vi "Split.vi"(2 "error in":errorcluster caption="错误输入（无错误）", 3 "ViewCtl":T1) -> (0 "error out":errorcluster caption="错误输出", 1 "StartArr":bool[](array[boolean]))   [LabVIEW 2013]
uses:
  Ctl/ViewCtl.ctl
  USBCAN/DevType.ctl
panel:
  # "ms"
  # "ms"
  # "s"
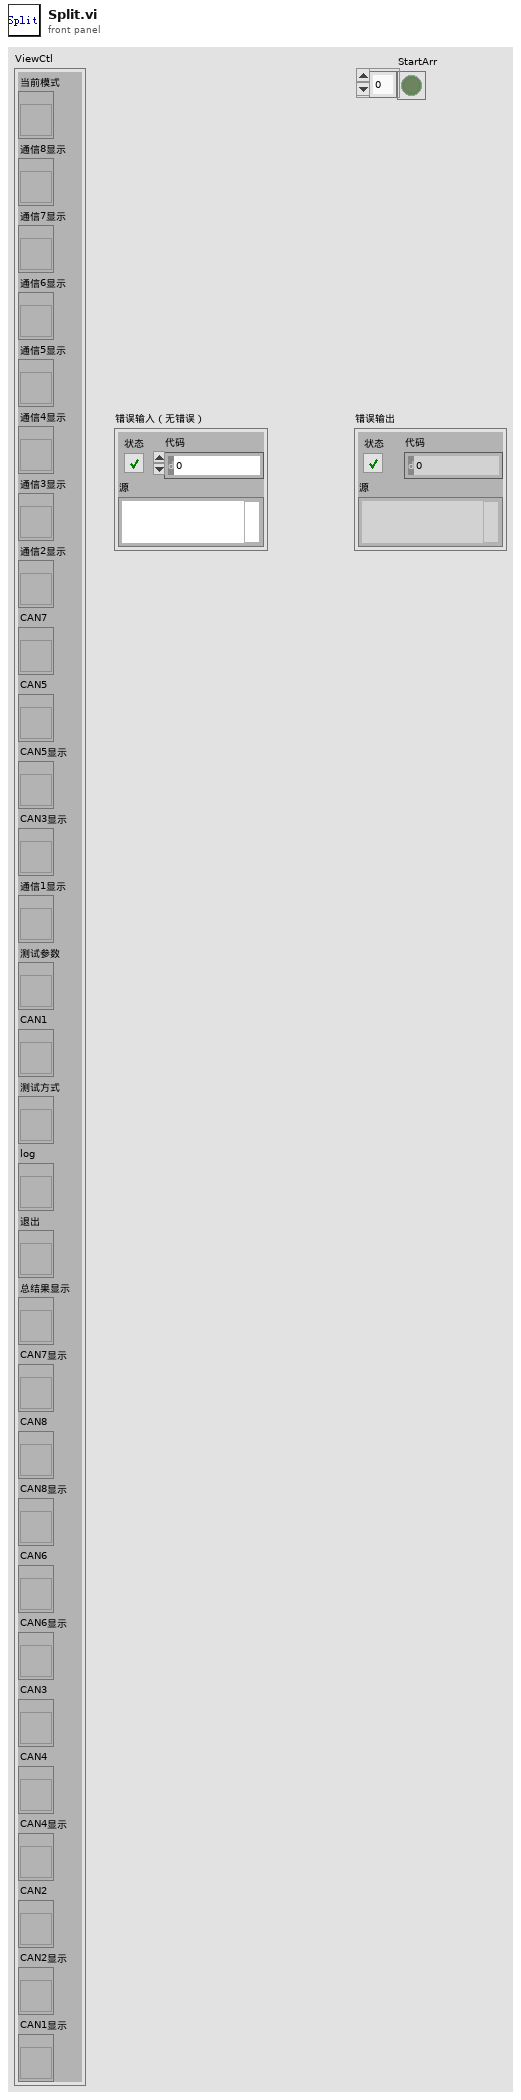
[diagram p1: front panel]
types:
  T1 = typedef "ViewCtl.ctl" = cluster{"当前模式":refnum<vi>, "通信8显示":refnum<vi>, "通信7显示":refnum<vi>, "通信6显示":refnum<vi>, "通信5显示":refnum<vi>, "通信4显示":refnum<vi>, "通信3显示":refnum<vi>, "通信2显示":refnum<vi>, "CAN7":refnum<vi>, "CAN5":refnum<vi>, "CAN5显示":refnum<vi>, "CAN3显示":refnum<vi>, "通信1显示":refnum<vi>, "测试参数":refnum<vi>, "CAN1":refnum<vi>, "测试方式":refnum<vi>, "log":refnum<vi>, "退出":refnum<vi>, "总结果显示":refnum<vi>, "CAN7显示":refnum<vi>, "CAN8":refnum<vi>, "CAN8显示":refnum<vi>, "CAN6":refnum<vi>, "CAN6显示":refnum<vi>, "CAN3":refnum<vi>, "CAN4":refnum<vi>, "CAN4显示":refnum<vi>, "CAN2":refnum<vi>, "CAN2显示":refnum<vi>, "CAN1显示":refnum<vi>}
  T2 = typedef "DevType.ctl" = u16
  T3 = cluster{"帧ID1":u32, "等待延时":u32, "间隔延时":u32, "总时间":u32, "总次数":u32, "发送数据1":string, "接收数据1":string, "发送数据2":string, "接收数据2":string, "CAN盒类型":T2, "帧ID2":u32, "同步启动个数":u8, "模式":enum16{"整体", "单个"}, "Baud":u8}
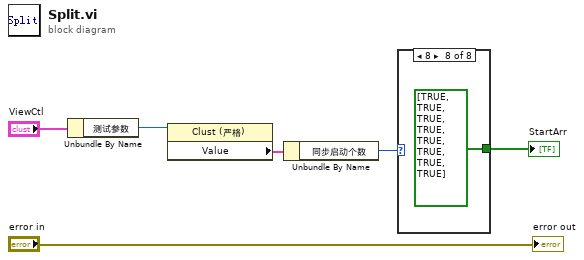
[diagram p0: block diagram]
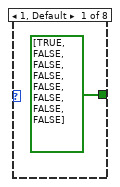
[diagram p2: hidden frame]
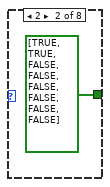
[diagram p3: hidden frame]
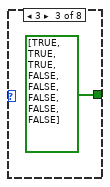
[diagram p4: hidden frame]
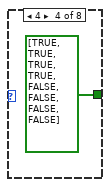
[diagram p5: hidden frame]
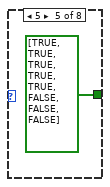
[diagram p6: hidden frame]
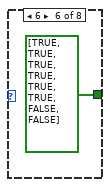
[diagram p7: hidden frame]
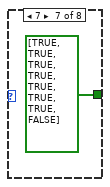
[diagram p8: hidden frame]
diagram:
  n1 = Unbundle By Name("ViewCtl") -> ("测试参数"=w5:refnum<vi>)
  n2 = property class="Clust (严格)"(reference=w5) -> ("Value"=w4:T3)  [unwired: 1 in, 2 out]
  n3 = Unbundle By Name(w4) -> ("同步启动个数"=w2:u8)
  n4 = case shown="8" w2 {
    tunnel: [bool[] [TRUE, FALSE, FALSE, FALSE, FALSE, FALSE, FALSE, FALSE] bool[] [TRUE, TRUE, FALSE, FALSE, FALSE, FALSE, FALSE, FALSE] bool[] [TRUE, TRUE, TRUE, FALSE, FALSE, FALSE, FALSE, FALSE] bool[] [TRUE, TRUE, TRUE, TRUE, FALSE, FALSE, FALSE, FALSE] bool[] [TRUE, TRUE, TRUE, TRUE, TRUE, FALSE, FALSE, FALSE] bool[] [TRUE, TRUE, TRUE, TRUE, TRUE, TRUE, FALSE, FALSE] bool[] [TRUE, TRUE, TRUE, TRUE, TRUE, TRUE, TRUE, FALSE] bool[] [TRUE, TRUE, TRUE, TRUE, TRUE, TRUE, TRUE, TRUE]] -> w1
    frame 1, Default {
    }
    frame 2 {
    }
    frame 3 {
    }
    frame 4 {
    }
    frame 5 {
    }
    frame 6 {
    }
    frame 7 {
    }
    frame 8 {
    }
  }
  "StartArr" <- w1
  "error out" <- "error in"
